vi "Saved Checker.vi"(1 "comp A":T1, 2 "comp B":T2) -> (0 "Unsaved":bool)   [LabVIEW 2018]
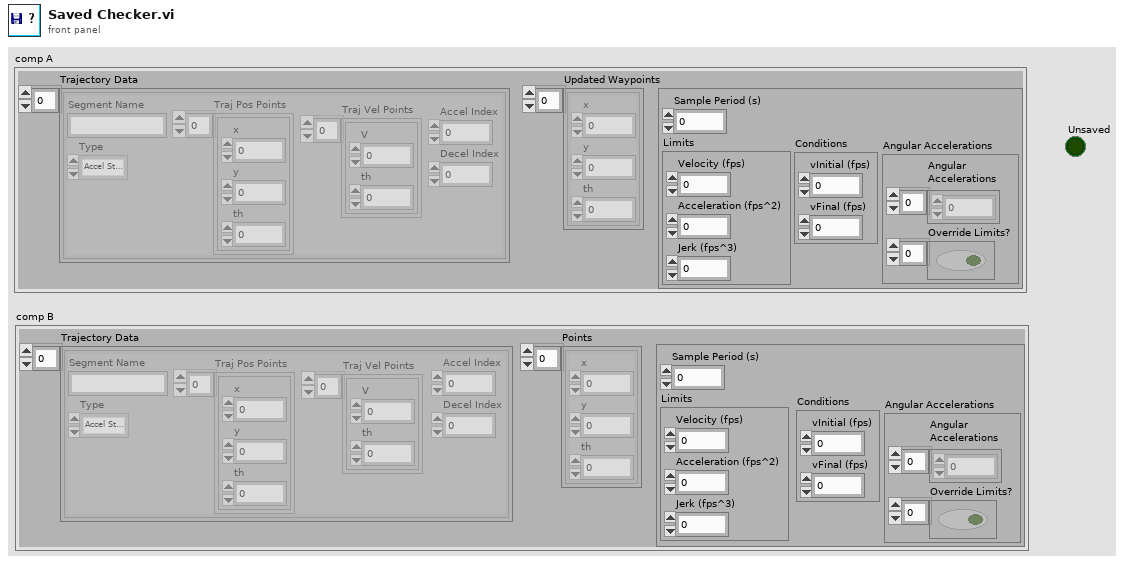
[diagram p1: front panel]
types:
  T1 = cluster{"Trajectory Data":cluster{"Segment Name":string, "Type":enum16{"Accel Straight", "Const Straight", "Blend", "Circle"}, "Traj Pos Points":cluster{"x":dbl, "y":dbl, "th":dbl}[], "Traj Vel Points":cluster{"V":dbl, "th":dbl}[], "Accel Index":i32, "Decel Index":i32}[], "Updated Waypoints":cluster{"x":dbl, "y":dbl, "th":dbl}[], cluster{"Sample Period (s)":dbl, "Limits":cluster{"Velocity (fps)":dbl, "Acceleration (fps^2)":dbl, "Jerk (fps^3)":dbl}, "Conditions":cluster{"vInitial (fps)":dbl, "vFinal (fps)":dbl}, "Angular Accelerations":cluster{"Angular \nAccelerations":dbl[], "Override Limits?":bool[]}}}
  T2 = cluster{"Trajectory Data":cluster{"Segment Name":string, "Type":enum16{"Accel Straight", "Const Straight", "Blend", "Circle"}, "Traj Pos Points":cluster{"x":dbl, "y":dbl, "th":dbl}[], "Traj Vel Points":cluster{"V":dbl, "th":dbl}[], "Accel Index":i32, "Decel Index":i32}[], "Points":cluster{"x":dbl, "y":dbl, "th":dbl}[], cluster{"Sample Period (s)":dbl, "Limits":cluster{"Velocity (fps)":dbl, "Acceleration (fps^2)":dbl, "Jerk (fps^3)":dbl}, "Conditions":cluster{"vInitial (fps)":dbl, "vFinal (fps)":dbl}, "Angular Accelerations":cluster{"Angular \nAccelerations":dbl[], "Override Limits?":bool[]}}}
  T3 = cluster{"Segment Name":string, "Type":enum16{"Accel Straight", "Const Straight", "Blend", "Circle"}, "Traj Pos Points":cluster{"x":dbl, "y":dbl, "th":dbl}[], "Traj Vel Points":cluster{"V":dbl, "th":dbl}[], "Accel Index":i32, "Decel Index":i32}[]
  T4 = cluster{"Sample Period (s)":dbl, "Limits":cluster{"Velocity (fps)":dbl, "Acceleration (fps^2)":dbl, "Jerk (fps^3)":dbl}, "Conditions":cluster{"vInitial (fps)":dbl, "vFinal (fps)":dbl}, "Angular Accelerations":cluster{"Angular \nAccelerations":dbl[], "Override Limits?":bool[]}}
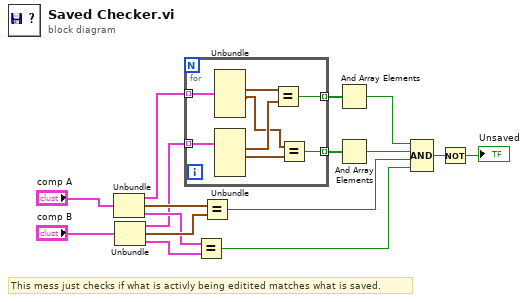
[diagram p0: block diagram]
diagram:
  # "This mess just checks if what is activly being editited matches what is saved."
  n1 = Unbundle("comp A") -> ("Trajectory Data"=w11:T3, "Updated Waypoints"=w14:cluster{"x":dbl, "y":dbl, "th":dbl}[], w12:T4)
  n2 = Unbundle("comp B") -> ("Trajectory Data"=w9:T3, "Points"=w13:cluster{"x":dbl, "y":dbl, "th":dbl}[], w10:T4)
  n3 = for {
    tunnel: w11 -> [w24] mode=indexing
    tunnel: w9 -> [w23] mode=indexing
    tunnel: [w18] -> w8 mode=indexing
    tunnel: [w17] -> w7 mode=indexing
    n4 = Unbundle(w24) -> ("Traj Pos Points"=w22:cluster{"x":dbl, "y":dbl, "th":dbl}[], "Traj Vel Points"=w19:cluster{"V":dbl, "th":dbl}[])  [unwired: 4 out]
    n5 = Unbundle(w23) -> ("Traj Pos Points"=w21:cluster{"x":dbl, "y":dbl, "th":dbl}[], "Traj Vel Points"=w20:cluster{"V":dbl, "th":dbl}[])  [unwired: 4 out]
    n6 = Equal?(x=w22, y=w21) -> (x = y?=w18:bool)
    n7 = Equal?(x=w19, y=w20) -> (x = y?=w17:bool)
  }
  n8 = Equal?(x=w12, y=w10) -> (x = y?=w3:bool)
  n9 = Equal?(x=w14, y=w13) -> (x = y?=w4:bool)
  n10 = And Array Elements(Boolean array=w8) -> (logical AND=w6:bool)
  n11 = And Array Elements(Boolean array=w7) -> (logical AND=w5:bool)
  n12 = Compound Arithmetic op=AND(w6, w5, w4, w3) -> (w2:bool)
  n13 = Not(x=w2) -> (.not. x?=→"Unsaved":bool)
